vi "Parse State Queue Empty Input String Performance Test.vi"() -> ()   [LabVIEW 2013]
panel:
  out "String":string
  out "Times Faster":dbl
  out "Waveform Chart":u32(graph)
  out "New":u32
  out "Old":u32
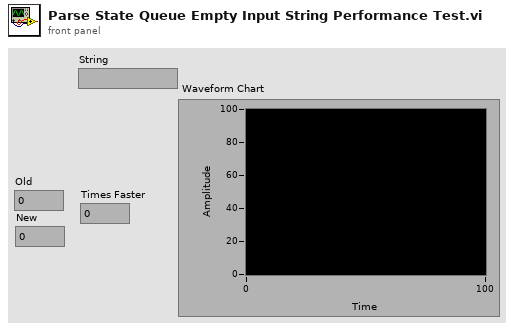
[diagram p1: front panel]
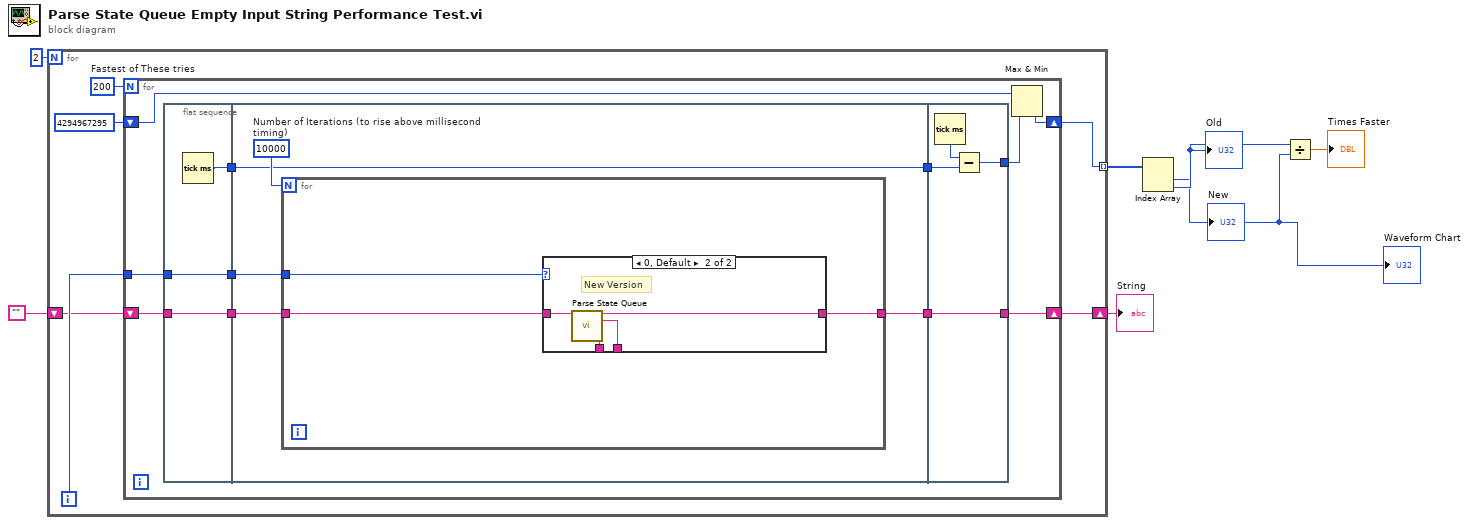
[diagram p0: block diagram]
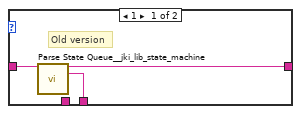
[diagram p2: hidden frame]
diagram:
  n1 = for {
    N: 2 -> [_]
    tunnel: [w10] -> w6 mode=indexing
    shift-right: [w9] -> w1
    shift-left: "" -> [w8]
    i -> [w13]
    w12 = 200  # Fastest of These tries
    n2 = for {
      N: w12 -> [_]
      tunnel: w13 -> [w21]
      shift-right: [w20] -> w10
      shift-left: u32 4294967295 -> [w18]
      shift-right: [w14] -> w9
      shift-left: w8 -> [w15]
      n3 = flat-sequence {
        tunnel: [w27] -> w24
        tunnel: w21 -> [w26]
        tunnel: [w26] -> w23
        tunnel: [w25] -> w16
        tunnel: w15 -> [w25]
        tunnel: w24 -> [w31]
        tunnel: [w31] -> w22
        tunnel: w23 -> [w30]
        tunnel: [w29] -> w17
        tunnel: w16 -> [w28]
        tunnel: w22 -> [w45]
        tunnel: [w44] -> w19
        tunnel: w17 -> [w43]
        tunnel: [w43] -> w14
        frame #0 {
          n4 = Tick Count (ms)() -> (millisecond timer value=w27:u32)
        }
        frame #1 {
          w32 = 10000  # Number of Iterations (to rise above millisecond timing)
          n5 = for {
            N: w32 -> [_]
            tunnel: w30 -> [w35]
            tunnel: [w34] -> w29
            tunnel: w28 -> [w33]
            n6 = case shown="0, Default" w35 {
              tunnel: w33 -> [w38 w42]
              tunnel: [w37 w41] -> _
              tunnel: [w36 w40] -> w34
              tunnel: [_ w39] -> _
              frame 1 {
                # "Old version"
                n7 = call <vilib>:"Parse State Queue__jki_lib_state_machine.vi"("State Queue"=w38) -> ("Remaining States"=w36:string, "Current State"=w37:string)  [unwired: 12 in, 1 out]
              }
              frame 0, Default {
                # "New Version"
                n8 = call "Parse State Queue.vi"("State Queue"=w42) -> ("Remaining States"=w40:string, "Current State"=w41:string, "Arguments"=w39:string)  [unwired: 12 in]
              }
            }
          }
        }
        frame #2 {
          n9 = Tick Count (ms)() -> (millisecond timer value=w46:u32)
          n10 = Subtract(x=w46, y=w45) -> (x-y=w44:u32)
        }
      }
      n11 = Max & Min(x=w18, y=w19) -> (min(x,y)=w20:u32)  [unwired: 1 out]
    }
  }
  "String" <- w1
  n12 = Index Array(array=w6) -> (element #1=w3:u32, element #2=w4:u32)  [unwired: 2 in]
  "Old" <- w4
  "New" <- w3
  "Waveform Chart" <- w3
  n13 = Divide(x=w4, y=w3) -> (x/y=→"Times Faster":dbl)
